vi "WSVCAP SHL Host TL I2C Write - Multiple Device - Common Data.vi"(0 "Sub Address":u8=20 format="%.0x", 5 "Data Out [U8]":u8=20 format="%.0x", 11 "error in":errorcluster, 12 "Log (T)":bool=TRUE, 13 "DUT Mask Array (All)":bool[][](array[boolean])=[[TRUE, TRUE, TRUE, TRUE, TRUE, TRUE, TRUE, TRUE, TRUE, TRUE, TRUE, TRUE, TRUE, TRUE, TRUE, TRUE, FALSE, FALSE, FALSE, FALSE, FALSE, FALSE, FALSE, FALSE, FALSE, FALSE, FALSE, FALSE, FALSE, FALSE, FALSE, FALSE], [TRUE, TRUE, TRUE, TRUE, TRUE, TRUE, TRUE, TRUE, TRUE, TRUE, TRUE, TRUE, TRUE, TRUE, TRUE, TRUE, FALSE, FALSE, FALSE, FALSE, FALSE, FALSE, FALSE, FALSE, FALSE, FALSE, FALSE, FALSE, FALSE, FALSE, FALSE, FALSE], [TRUE, TRUE, TRUE, TRUE, TRUE, TRUE, TRUE, TRUE, TRUE, TRUE, TRUE, TRUE, TRUE, TRUE, TRUE, TRUE, TRUE, FALSE, FALSE, FALSE, FALSE, FALSE, TRUE, FALSE, FALSE, FALSE, FALSE, FALSE, FALSE, FALSE, FALSE, TRUE], [FALSE, FALSE, FALSE, FALSE, FALSE, FALSE, FALSE, FALSE, FALSE, FALSE, FALSE, FALSE, FALSE, FALSE, FALSE, FALSE, TRUE, FALSE, FALSE, FALSE, FALSE, FALSE, TRUE, FALSE, FALSE, FALSE, FALSE, FALSE, FALSE, FALSE, FALSE, TRUE]], 14 "DUT Mask Mode (All)":T1=enum."All") -> (15 "error out":errorcluster)   [LabVIEW 2012]
uses:
  Type Defs/WSVCAP SHL I2C DUT Mask Mode Enum.ctl
panel:
  out "C3 Data Out":u8[](array[numeric]) format="%.0x"
  out "Socket Mask":u64=1 format="%02x"
  out "C2 Data Out":u8[](array[numeric]) format="%.0x"
  out "C1 Data Out":u8[](array[numeric]) format="%.0x"
  # "DUT 01"
  # "DUT 02"
  # "DUT 03"
  # "DUT 04"
  # "DUT 05"
  # "DUT 06"
  # "DUT 07"
  # "DUT 08"
  # "DUT 09"
  # "DUT 10"
  # "DUT 11"
  # "DUT 12"
  # "DUT 13"
  # "DUT 14"
  # "DUT 15"
  # "DUT 16"
  # "C1"
  # "C2"
  # "C3"
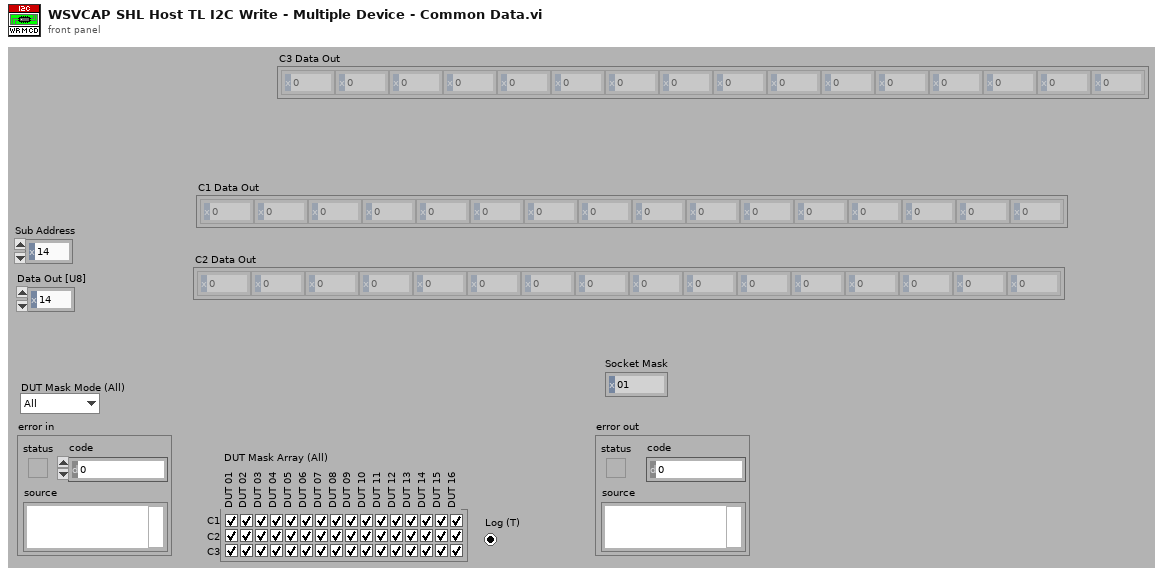
[diagram p1: front panel]
types:
  T1 = typedef "WSVCAP SHL I2C DUT Mask Mode Enum.ctl" = enum16{"Custom", "C1", "C2", "C3", "All"}
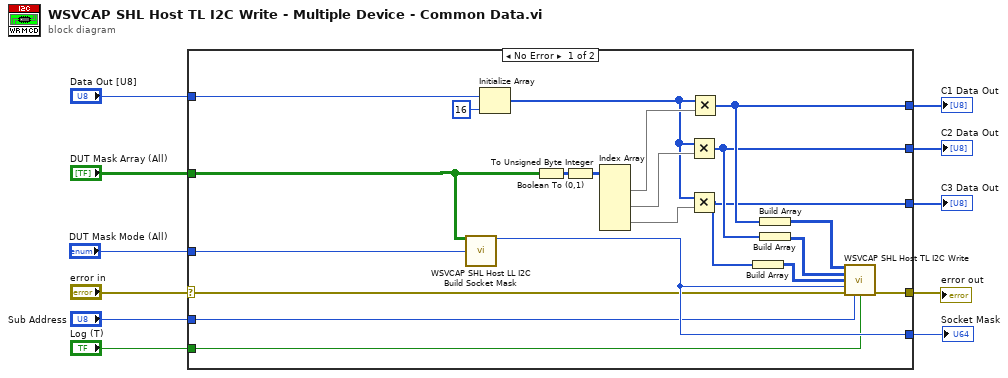
[diagram p0: block diagram]
diagram:
  n1 = case shown="No Error" "error in" {
    selector: "error in" -> [w20 w33]
    tunnel: [w32 w33] -> w11
    tunnel: "Sub Address" -> [w15 _]
    tunnel: "Data Out [U8]" -> [w27 _]
    tunnel: [w21 _] -> w7
    tunnel: [w22 _] -> w6
    tunnel: [w29 _] -> w5
    tunnel: "DUT Mask Array (All)" -> [w13 _]
    tunnel: "Log (T)" -> [w19 _]
    tunnel: [w14 _] -> w2
    tunnel: "DUT Mask Mode (All)" -> [w12 _]
    frame No Error {
      n2 = call "WSVCAP SHL Host LL I2C Build Socket Mask.vi"("DUT Mask Array"=w13, "DUT Mask Mode (Custom)"=w12) -> ("Socket Mask [U64]"=w29:u64)  [unwired: 12 in, 1 out]
      n3 = Initialize Array(w27, 16 ("dimension size")) -> (w18:u8[])
      n4 = Boolean To (0,1)(Boolean=w13) -> (0, 1=w28:i16[][])
      n5 = To Unsigned Byte Integer(number=w28) -> (unsigned 8bit integer=w23:u8[][])
      n6 = Index Array(array=w23) -> (element #1=w25:u8[], element #2=w24:u8[], element #3=w17:u8[])  [unwired: 6 in]
      n7 = Multiply(x=w18, y=w24) -> (x*y=w21:u8[])
      n8 = Multiply(x=w18, y=w17) -> (x*y=w14:u8[])
      n9 = Multiply(x=w18, y=w25) -> (x*y=w22:u8[])
      n10 = Build Array(w14) -> (w16:u8[][])
      n11 = Build Array(w22) -> (w31:u8[][])
      n12 = Build Array(w21) -> (w30:u8[][])
      n13 = call "WSVCAP SHL Host TL I2C Write.vi"("C1 Data Out"=w31, "C2 Data Out"=w30, "C3 Data Out"=w16, "Socket Mask [U64]"=w29, "error in"=w20, "Sub Address"=w15, "Log (T)"=w19) -> ("error out"=w32:errorcluster)  [unwired: 8 in]
    }
    frame Error {
    }
  }
  "error out" <- w11
  "C1 Data Out" <- w6
  "C2 Data Out" <- w7
  "Socket Mask" <- w5
  "C3 Data Out" <- w2
